vi "specrugram_params_set.vi"(6 "fs":dbl, 7 "center frequncy":dbl, 8 "file size":i64, 9 "reading time frame (sec)":dbl, 10 "fft size in power of  in":i32, 11 "?":refnum<vi>) -> (0 "number of plots":ext, 1 "time in file":dbl, 2 "fft size":ext, 3 "sampels per plot":ext, 4 "time per plot":ext)   [LabVIEW 2021]
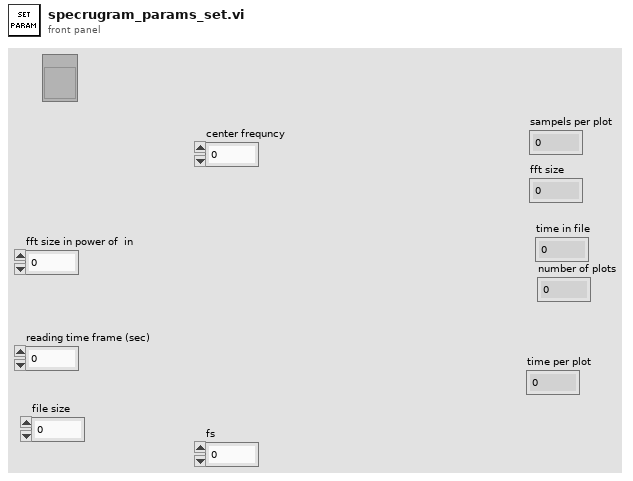
[diagram p1: front panel]
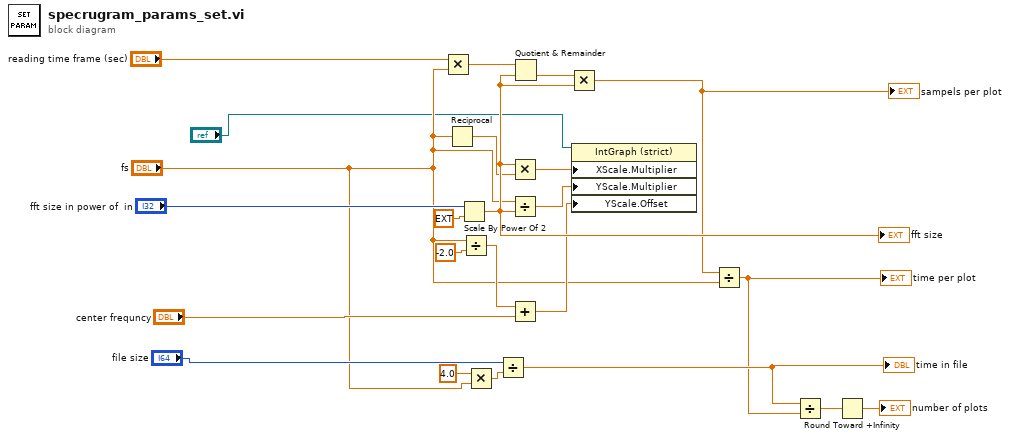
[diagram p0: block diagram]
diagram:
  n1 = Multiply(x="reading time frame (sec)", y="fs") -> (x*y=w15:dbl)
  n2 = Reciprocal(x="fs") -> (1/x=w18:dbl)
  n3 = Scale By Power Of 2(n="fft size in power of  in", x=ext 1.0) -> (x*2^n=w23:ext)
  "fft size" <- w23
  n4 = Divide(x="fs", y=-2.0) -> (x/y=w20:dbl)
  n5 = Multiply(x=4.0, y="fs") -> (x*y=w8:dbl)
  n6 = Divide(x="file size", y=w8) -> (x/y=w5:dbl)
  "time in file" <- w5
  n7 = Multiply(x=w23, y=w18) -> (x*y=w13:ext)
  n8 = Divide(x="fs", y=w23) -> (x/y=w12:ext)
  n9 = Add(x=w20, y="center frequncy") -> (x+y=w11:dbl)
  n10 = Quotient & Remainder(x=w15, y=w23) -> (floor(x/y)=w22:ext)  [unwired: 1 out]
  n11 = Multiply(x=w22, y=w23) -> (x*y=w10:ext)
  "sampels per plot" <- w10
  n12 = property on="Property Node" class="IntGraph (strict)"(reference="?", "XScale.Multiplier"=w13, "YScale.Multiplier"=w12, "YScale.Offset"=w11) -> ()  [unwired: 1 in, 2 out]
  n13 = Divide(x=w10, y="fs") -> (x/y=w4:ext)
  "time per plot" <- w4
  n14 = Divide(x=w5, y=w4) -> (x/y=w7:ext)
  n15 = Round Toward +Infinity(x=w7) -> (ceil(x): smallest int >= x=→"number of plots":ext)
